vi "Config.vi"(8 "error in (no error)":errorcluster, 10 "Setting":variant, 11 "Tektronix Scope in":refnum<class "Tektronix MSO5.lvclass">) -> (0 "error out":errorcluster, 3 "Tektronix Scope out":refnum<class "Tektronix MSO5.lvclass">)   [LabVIEW 2025, in "Scope.lvlib" / "Tektronix MSO5.lvclass"]
uses:
  Tektronix MSO5.lvclass
  Tektronix MSO5.lvclass/Tektronix MSO5.ctl
  <instrlib>/Tektronix MSO5 Series/Drivers/Tektronix MSO5X Series.lvlib
  Scope configuration/Scope configuration.lvclass
  Scope Channel/Scope Channel.lvclass
  Scope Channel configuration/Scope Channel configuration.lvclass
  <instrlib>/Tektronix MSO5 Series/Utilities/MS058LP Library.lvlib
  <instrlib>/niScope/Controls/niScope vertical coupling.ctl
  <instrlib>/niScope/Controls/niScope trigger coupling.ctl
  <instrlib>/Tektronix MSO5 Series/Utilities/Trigger Type.ctl
  Users/Public/Documents/Sandia National Labs/TSS Plugin/Abstract Engine.lvlibp/Plugin/Abstract/Abstract Instrument/Channel.ctl
  Users/Public/Documents/Sandia National Labs/TSS Plugin/Abstract Engine.lvlibp/Plugin/Abstract/Abstract Instrument/Abstract Instrument.lvclass
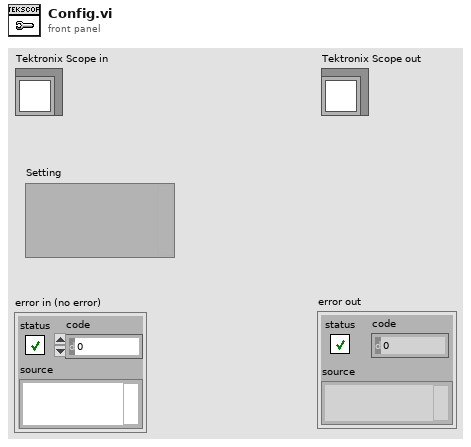
[diagram p1: front panel]
types:
  T1 = typedef "MS058LP Library.lvlib/Trigger Type.ctl" = enum16{"Immediate", "Software", "Analog Edge - Positive", "Analog Edge - Negative", "Digital Edge - Positive", "Digital Edge - Negative", "Window - Entering", "Window - Leaving", "Hysteresis - Positive", "Hysteresis - Negative"}
  T2 = typedef "niScope trigger coupling.ctl" = u16
  T3 = cluster{"Sampling Rate":dbl, "Number of Samples":i32, "Trigger Type":T1, "Trigger Coupling":T2, "Trigger Source":string, "Trigger Level 1 (V)":dbl, "Trigger Level 2 (V)":dbl, "Pretrigger (%)":dbl, "Acquisition Complete":bool}
  T4 = typedef "Abstract Engine.lvlibp/Abstract Instrument.lvclass/Channel.ctl" = cluster{"Alias":string, "DataType":enum16{"Anaolg Input", "Waveform"}, "Unit":enum16{"---", "V", "A", "Ohm", "Hz", "uF", "degC", "deg"}, "Upper limit":dbl, "Lower limit":dbl, "Measurement":variant}
  T5 = typedef "niScope vertical coupling.ctl" = i32
  T6 = cluster{"Gain":dbl, "Offset":dbl, "Units":string, "V. Range":dbl, "V. Offset":dbl, "Attenuation":dbl, "Coupling":T5, "Impedance":u32}
  T7 = typedef "Abstract Engine.lvlibp/Channel configuration.lvclass/Default Channel.ctl" = cluster{"Address":string, "SW Alias":string, "Enabled":bool, "Type":string, "Description":string}
  T8 = typedef "Scope.lvlib/Scope Channel configuration.lvclass/Scope Channel Setting.ctl" = cluster{"Gain":u32, "Offset":u32, "Vertical Range":dbl, "Vertical Offset":dbl, "Unit":string, "Attenuation":dbl, "Vertical Coupling":string, "Impedance":string, "Auto Setup":bool}
  T9 = typedef "Scope.lvlib/Scope configuration.lvclass/Scope Instrument Setting.ctl" = cluster{"Sampling Rate":dbl, "Number of Samples":u32, "Type":string, "Pretrigger":dbl, "Source":string, "Level 1":dbl, "Level 2":dbl, "Trigger Coupling":string, "TrigDest":string, "Group":string}
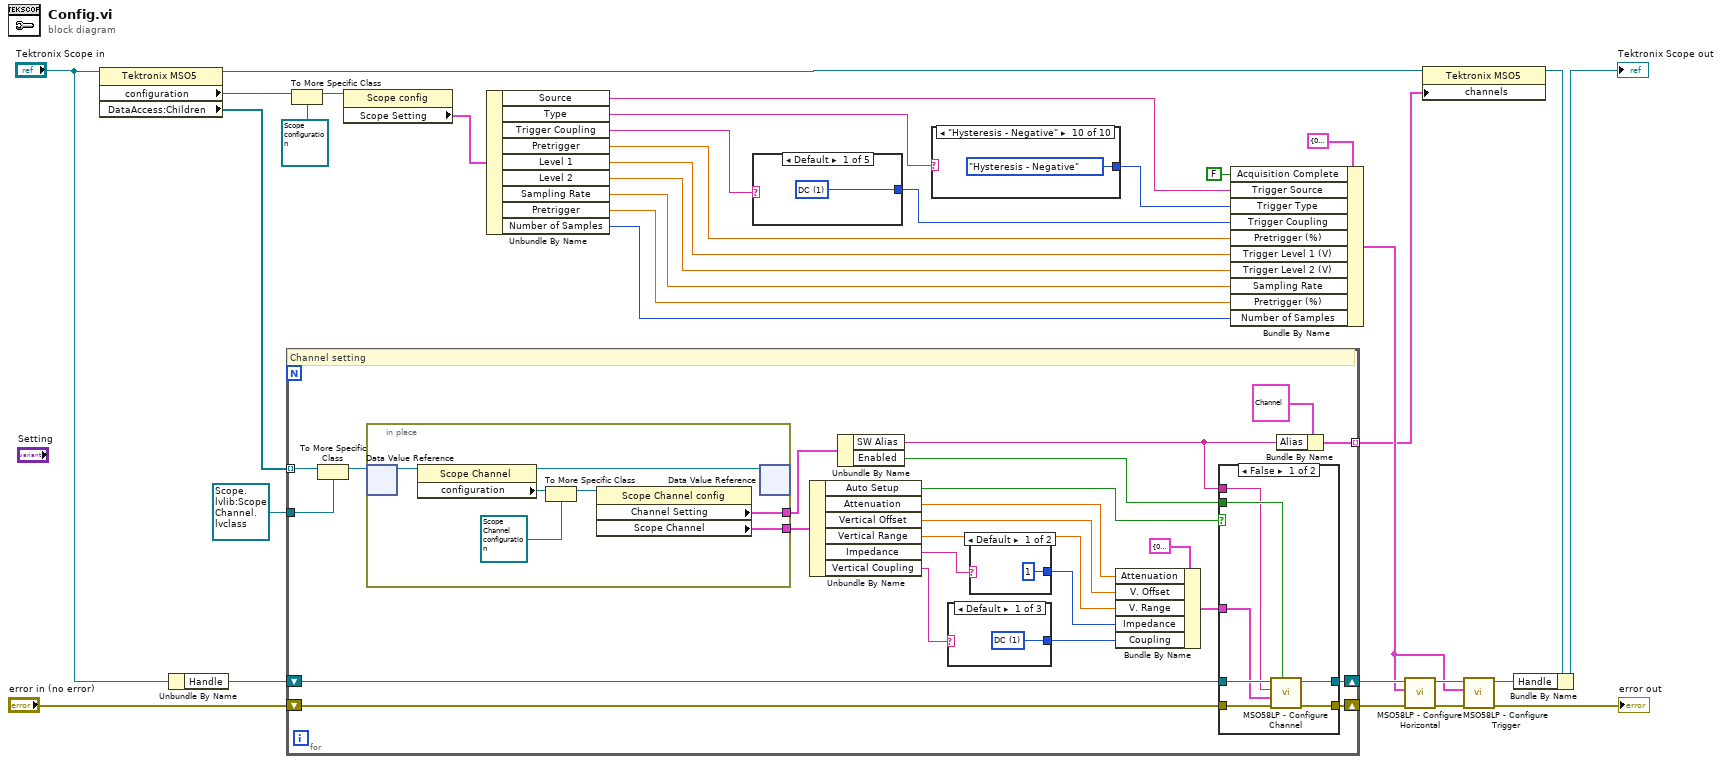
[diagram p0: block diagram]
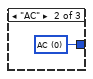
[diagram p2: hidden frame]
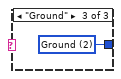
[diagram p3: hidden frame]
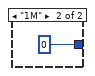
[diagram p4: hidden frame]
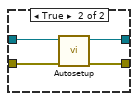
[diagram p5: hidden frame]
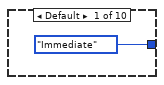
[diagram p6: hidden frame]
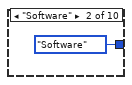
[diagram p7: hidden frame]
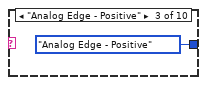
[diagram p8: hidden frame]
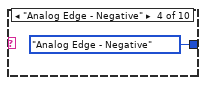
[diagram p9: hidden frame]
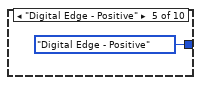
[diagram p10: hidden frame]
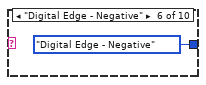
[diagram p11: hidden frame]
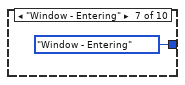
[diagram p12: hidden frame]
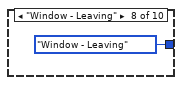
[diagram p13: hidden frame]
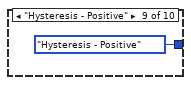
[diagram p14: hidden frame]
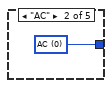
[diagram p15: hidden frame]
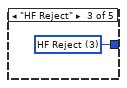
[diagram p16: hidden frame]
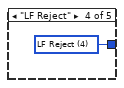
[diagram p17: hidden frame]
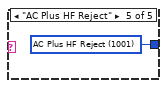
[diagram p18: hidden frame]
diagram:
  n1 = property class="Tektronix MSO5"(reference="Tektronix Scope in") -> (reference out=w31:refnum<class "Tektronix MSO5.lvclass">, "configuration"=w28:refnum<class "CEF_serializable configuration.lvclass">, "DataAccess:Children"=w26:refnum<data-value>[])  [unwired: 1 in, 1 out]
  n2 = Unbundle By Name("Tektronix Scope in") -> ("Handle"=w29:refnum<visa-resource-name>)
  n3 = for {
    tunnel: [w35] -> w1 mode=indexing
    shift-right: [w46] -> w23
    shift-left: "error in (no error)" -> [w52]
    shift-right: [w47] -> w22
    shift-left: w29 -> [w53]
    tunnel: w26 -> [w56] mode=indexing
    tunnel: refnum<data-value> refnum ("data value reference") -> [w54]
    # "Channel setting"
    n4 = To More Specific Class(target class=w54, reference=w56) -> (specific class reference=w55:refnum<data-value>)  [unwired: 1 in, 1 out]
    n5 = in-place {
      in-place-border: [w58] -> w45
      in-place-border: [w57] -> w43
      # "Initialize the front panel controls when loaded"
      n6 = in-place-dvr #1(w55) -> (w63:refnum<class "Scope Channel.lvclass">)  [unwired: 1 out]
      n7 = property class="Scope Channel"(reference=w63) -> (reference out=w62:refnum<class "Scope Channel.lvclass">, "configuration"=w61:refnum<class "CEF_serializable configuration.lvclass">)  [unwired: 1 in, 1 out]
      n8 = To More Specific Class(target class=refnum<class "Scope Channel configuration.lvclass"> refnum ("Scope.lvlib:Scope Channel configuration.lvclass"), reference=w61) -> (specific class reference=w60:refnum<class "Scope Channel configuration.lvclass">)  [unwired: 1 in, 1 out]
      n9 = property class="Scope Channel config"(reference=w60) -> ("Channel Setting"=w58:T7, "Scope Channel"=w57:T8)  [unwired: 1 in, 2 out]
      n10 = in-place-dvr #1(w62) -> ()  [unwired: 2 out]
    }
    n11 = Unbundle By Name(w43) -> ("Auto Setup"=w42:bool, "Attenuation"=w41:dbl, "Vertical Offset"=w40:dbl, "Vertical Range"=w39:dbl, "Impedance"=w38:string, "Vertical Coupling"=w37:string)
    n12 = Unbundle By Name(w45) -> ("SW Alias"=w36:string, "Enabled"=w44:bool)
    n13 = case shown="Default" w37 {
      tunnel: [w64 w65 w66] -> w48
      frame Default {
        w64 = T5 1 items=["AC", "DC", "Ground"] ("Coupling")
      }
      frame "AC" {
        w65 = T5 0 items=["AC", "DC", "Ground"] ("Coupling")
      }
      frame "Ground" {
        w66 = T5 2 items=["AC", "DC", "Ground"] ("Coupling")
      }
    }
    n14 = case shown="Default" w38 {
      tunnel: [u32 1 ("Impedance") u32 0 ("Impedance")] -> w49
      frame Default {
      }
      frame "1M" {
      }
    }
    n15 = Bundle By Name(cluster=T6 {"Gain"=0.0, "Offset"=0.0, "Units"="", "V. Range"=0.0, "V. Offset"=0.0, "Attenuation"=0.0, "Coupling"=1, "Impedance"=0} ("Channel Info"), "Attenuation"=w41, "V. Offset"=w40, "V. Range"=w39, "Impedance"=w49, "Coupling"=w48) -> (w50:T6)
    n16 = case shown="False" w42 {
      tunnel: w53 -> [w75 w79]
      tunnel: [w74 w78] -> w47
      tunnel: w52 -> [w72 w77]
      tunnel: [w73 w76] -> w46
      tunnel: w50 -> [w71 _]
      tunnel: w36 -> [w69 _]
      tunnel: w44 -> [w70 _]
      frame False {
        n17 = call <instrlib>:"MSO58LP - Configure Channel.vi"("Enabled (T: Enable)"=w70, "Error In"=w72, "Channel Info"=w71, "Channel"=w69, "Visa In"=w75) -> ("Error out"=w73:errorcluster, "VISA Out"=w74:refnum<visa-resource-name>)  [unwired: 4 in, 1 out]
      }
      frame True {
        n18 = call <instrlib>:"Autosetup.vi"("error in (no error)"=w77, "VISA resource name"=w79) -> ("error out"=w76:errorcluster, "VISA resource name out"=w78:refnum<visa-resource-name>)  [unwired: 8 in]
      }
    }
    n19 = Bundle By Name(cluster=T4 {"Alias"="ch0", "DataType"=enum."Anaolg Input", "Unit"=enum."V", "Upper limit"=10.0, "Lower limit"=-10.0, "Measurement"=variant} ("Channel"), "Alias"=w36) -> (w35:T4)
  }
  n20 = To More Specific Class(target class=refnum<class "Scope configuration.lvclass"> refnum ("Scope.lvlib:Scope configuration.lvclass"), reference=w28) -> (specific class reference=w27:refnum<class "Scope configuration.lvclass">)  [unwired: 1 in, 1 out]
  n21 = property class="Scope config"(reference=w27) -> ("Scope Setting"=w3:T9)  [unwired: 1 in, 2 out]
  n22 = Unbundle By Name(w3) -> ("Source"=w8:string, "Type"=w5:string, "Trigger Coupling"=w9:string, "Pretrigger"=w12:dbl, "Level 1"=w13:dbl, "Level 2"=w14:dbl, "Sampling Rate"=w18:dbl, "Pretrigger"=w20:dbl, "Number of Samples"=w19:u32)
  n23 = case shown="Default" w9 {
    tunnel: [w80 w81 w82 w83 w84] -> w10
    frame Default {
      w80 = T2 1 items=["AC"=0, "DC"=1, "HF Reject"=3, "LF Reject"=4, "AC Plus HF Reject"=1001] ("Trigger Coupling")
    }
    frame "AC" {
      w81 = T2 0 items=["AC"=0, "DC"=1, "HF Reject"=3, "LF Reject"=4, "AC Plus HF Reject"=1001] ("Trigger Coupling")
    }
    frame "HF Reject" {
      w82 = T2 3 items=["AC"=0, "DC"=1, "HF Reject"=3, "LF Reject"=4, "AC Plus HF Reject"=1001] ("Trigger Coupling")
    }
    frame "LF Reject" {
      w83 = T2 4 items=["AC"=0, "DC"=1, "HF Reject"=3, "LF Reject"=4, "AC Plus HF Reject"=1001] ("Trigger Coupling")
    }
    frame "AC Plus HF Reject" {
      w84 = T2 1001 items=["AC"=0, "DC"=1, "HF Reject"=3, "LF Reject"=4, "AC Plus HF Reject"=1001] ("Trigger Coupling")
    }
  }
  n24 = case shown="\"Hysteresis - Negative\"" w5 {
    tunnel: [Trigger_Type."Immediate" ("Trigger Type") Trigger_Type."Software" ("Trigger Type") Trigger_Type."Analog Edge - Positive" ("Trigger Type") Trigger_Type."Analog Edge - Negative" ("Trigger Type") Trigger_Type."Digital Edge - Positive" ("Trigger Type") Trigger_Type."Digital Edge - Negative" ("Trigger Type") Trigger_Type."Window - Entering" ("Trigger Type") Trigger_Type."Window - Leaving" ("Trigger Type") Trigger_Type."Hysteresis - Positive" ("Trigger Type") Trigger_Type."Hysteresis - Negative" ("Trigger Type")] -> w4
    frame Default {
    }
    frame "Software" {
    }
    frame "Analog Edge - Positive" {
    }
    frame "Analog Edge - Negative" {
    }
    frame "Digital Edge - Positive" {
    }
    frame "Digital Edge - Negative" {
    }
    frame "Window - Entering" {
    }
    frame "Window - Leaving" {
    }
    frame "Hysteresis - Positive" {
    }
    frame "Hysteresis - Negative" {
    }
  }
  n25 = Bundle By Name(cluster=T3 {"Sampling Rate"=0.0, "Number of Samples"=0, "Trigger Type"=enum."Immediate", "Trigger Coupling"=1, "Trigger Source"="", "Trigger Level 1 (V)"=0.0, "Trigger Level 2 (V)"=0.0, "Pretrigger (%)"=0.0, "Acquisition Complete"=FALSE} ("Horizontal"), "Acquisition Complete"=FALSE, "Trigger Source"=w8, "Trigger Type"=w4, "Trigger Coupling"=w10, "Pretrigger (%)"=w12, "Trigger Level 1 (V)"=w13, "Trigger Level 2 (V)"=w14, "Sampling Rate"=w18, "Pretrigger (%)"=w20, "Number of Samples"=w19) -> (w15:T3)
  n26 = call <instrlib>:"MSO58LP - Configure Horizontal.vi"("Error In"=w23, "Horizontal"=w15, "Visa In"=w22) -> ("Error out"=w17:errorcluster, "VISA Out"=w16:refnum<visa-resource-name>)  [unwired: 7 in]
  n27 = property class="Tektronix MSO5"(reference=w31, "channels"=w1) -> (reference out=w2:refnum<class "Tektronix MSO5.lvclass">)  [unwired: 1 in, 1 out]
  n28 = call <instrlib>:"MSO58LP - Configure Trigger.vi"("error in"=w17, "Horizontal"=w15, "VISA In"=w16) -> ("error out"=→"error out":errorcluster, "VISA Out"=w6:refnum<visa-resource-name>)  [unwired: 7 in]
  n29 = Bundle By Name(cluster=w2, "Handle"=w6) -> (→"Tektronix Scope out":refnum<class "Tektronix MSO5.lvclass">)
